vi "PH_IEEE1394Camera.get Cam Attribute.vi"(0 "IMAQ1394 Session In":T4, 1 "Cam Attribute Name":string, 2 "Attribute Information Array":T3(array[cluster]), 5 "Cam Error in":errorcluster) -> (14 "IMAQ1394 Session Out":T4, 15 "Attribute read?":bool, 16 "Cam Attribute Value":T1, 19 "Cam Error out":errorcluster)   [LabVIEW 2014, in "PH_IEEE1394Camera.lvlib"]
doc: "This VI gets a camera attribute."
uses:
  PH_IEEE1394Camera.lvlib
  <vilib>/userdefined/High Color/IMAQdx.ctl
  <vilib>/vision/driver/IMAQdx.llb/IMAQdx Attribute Type.ctl
  PH_IEEE1394Camera.Cam Attribute.ctl
  <resource>/objmgr/imaqdx.rc
  <vilib>/vision/driver/NI_Vision_Acquisition_Software.lvlib
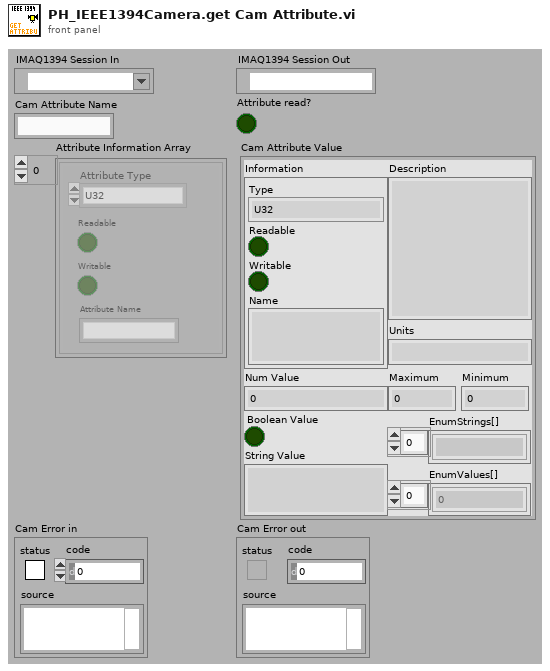
[diagram p1: front panel]
types:
  T1 = typedef "PH_IEEE1394Camera.lvlib/PH_IEEE1394Camera.Cam Attribute.ctl" = cluster{"Information":cluster{"Type":T2, "Readable":bool, "Writable":bool, "Name":string}, "Num Value":dbl, "String Value":string, "Maximum":dbl, "Minimum":dbl, "Units":string, "Description":string, "EnumStrings[]":string[], "EnumValues[]":u32[], "Boolean Value":bool}
  T2 = typedef "NI_Vision_Acquisition_Software.lvlib/IMAQdx Attribute Type.ctl" = enum32{"U32", "I64", "DBL", "String", "Enum", "Bool", "Command"}
  T3 = cluster{"Attribute Type":T2, "Readable":bool, "Writable":bool, "Attribute Name":string}[]
  T4 = typedef "IMAQdx.ctl" = refnum<k21>
  T5 = cluster{"Attribute Type":T2, "Readable":bool, "Writable":bool, "Attribute Name":string}
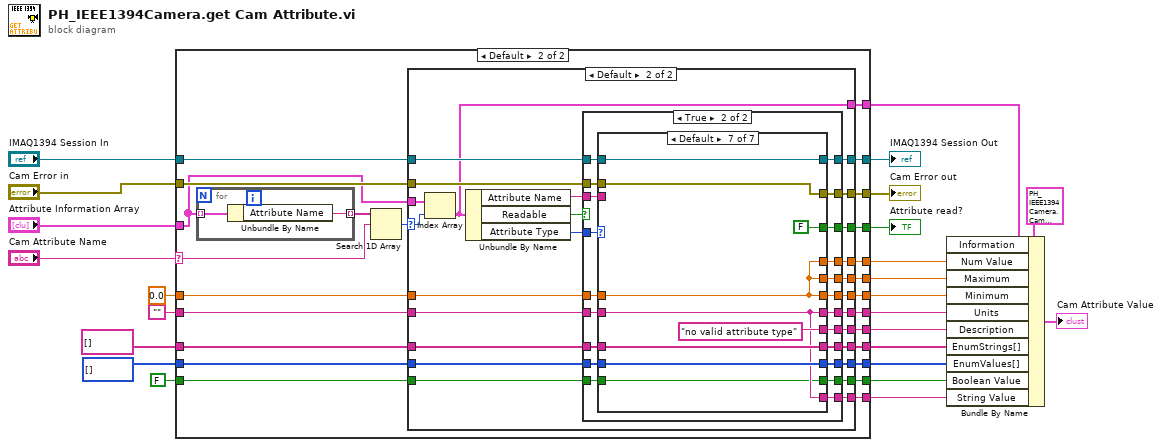
[diagram p0: block diagram]
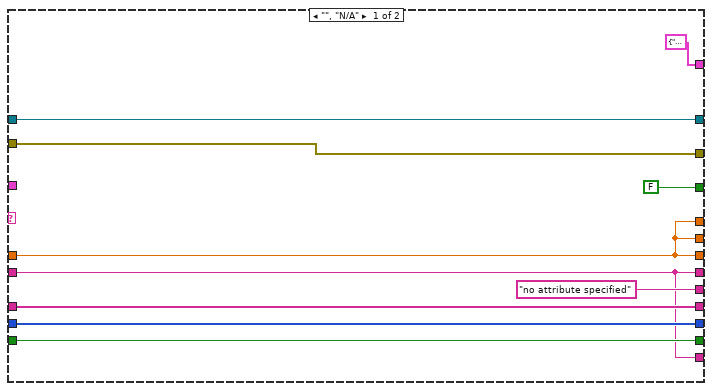
[diagram p2: hidden frame]
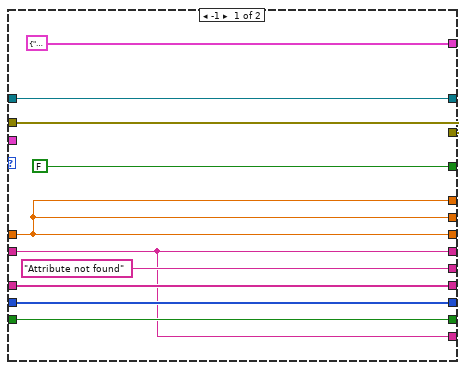
[diagram p3: hidden frame]
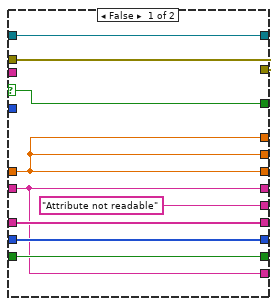
[diagram p4: hidden frame]
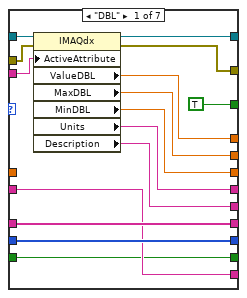
[diagram p5: hidden frame]
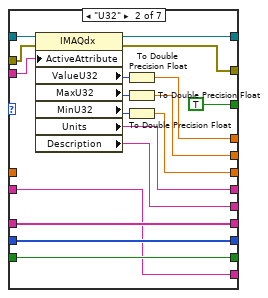
[diagram p6: hidden frame]
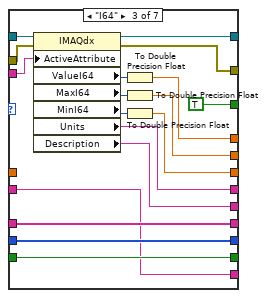
[diagram p7: hidden frame]
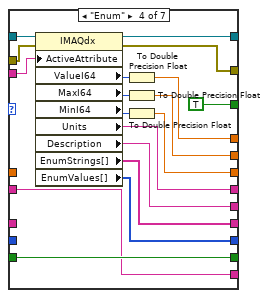
[diagram p8: hidden frame]
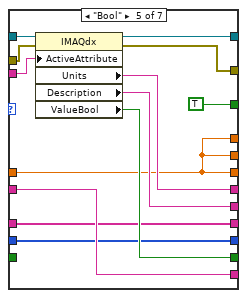
[diagram p9: hidden frame]
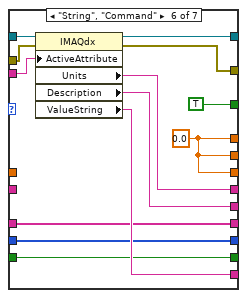
[diagram p10: hidden frame]
diagram:
  n1 = case shown="Default" "Cam Attribute Name" {
    selector: "Cam Attribute Name" -> [_ w54]
    tunnel: [w34 w58] -> w24
    tunnel: [w33 w57] -> w23
    tunnel: "Cam Error in" -> [w33 w56]
    tunnel: "IMAQ1394 Session In" -> [w34 w53]
    tunnel: [FALSE w55] -> w20
    tunnel: [w29 w52] -> w15
    tunnel: [w29 w51] -> w14
    tunnel: [w29 w50] -> w13
    tunnel: [w25 w49] -> w12
    tunnel: ["no attribute specified" w48] -> w11
    tunnel: [w28 w47] -> w10
    tunnel: [w27 w46] -> w9
    tunnel: [w26 w45] -> w8
    tunnel: [w25 w44] -> w7
    tunnel: "Attribute Information Array" -> [_ w43]
    tunnel: [T5 {"Attribute Type"=enum."U32", "Readable"=FALSE, "Writable"=FALSE, "Attribute Name"=""} ("Attribute Information") w40] -> w16
    tunnel: 0.0 ("ValueDBL") -> [w29 w39]
    tunnel: "" -> [w25 w38]
    tunnel: string[] [] ("EnumStrings[] 2") -> [w28 w37]
    tunnel: u32[] [] ("EnumValues[]") -> [w27 w36]
    tunnel: FALSE ("ValueBool") -> [w26 w35]
    frame "", "N/A" {
    }
    frame Default {
      n2 = for {
        tunnel: w43 -> [w229] mode=indexing
        tunnel: [w228] -> w42 mode=indexing
        n3 = Unbundle By Name(w229) -> ("Attribute Name"=w228:string)
      }
      n4 = Search 1D Array(1D array=w42, element=w54) -> (index of element=w41:i32)  [unwired: 1 in]
      n5 = case shown="Default" w41 {
        selector: w41 -> [_ w88]
        tunnel: [w67 w93] -> w58
        tunnel: w56 -> [w68 w92]
        tunnel: [w68 w91] -> w57
        tunnel: w53 -> [w67 w90]
        tunnel: w43 -> [_ w89]
        tunnel: [FALSE w85] -> w55
        tunnel: [w64 w83] -> w52
        tunnel: [w64 w82] -> w51
        tunnel: [w64 w81] -> w50
        tunnel: [w59 w80] -> w49
        tunnel: ["Attribute not found" w79] -> w48
        tunnel: [w62 w78] -> w47
        tunnel: [w61 w77] -> w46
        tunnel: [w60 w76] -> w45
        tunnel: [w59 w75] -> w44
        tunnel: [T5 {"Attribute Type"=enum."U32", "Readable"=FALSE, "Writable"=FALSE, "Attribute Name"=""} ("Attribute Information") w74] -> w40
        tunnel: w37 -> [w62 w73]
        tunnel: w36 -> [w61 w72]
        tunnel: w38 -> [w59 w71]
        tunnel: w39 -> [w64 w70]
        tunnel: w35 -> [w60 w69]
        frame -1 {
        }
        frame Default {
          n6 = Index Array(array=w89, index=w88) -> (element=w74:T5)
          n7 = Unbundle By Name(w74) -> ("Attribute Name"=w87:string, "Readable"=w86:bool, "Attribute Type"=w84:T2)
          n8 = case shown="True" w86 {
            selector: w86 -> [w100 _]
            tunnel: [w102 w123] -> w93
            tunnel: w92 -> [w101 w122]
            tunnel: [w101 w121] -> w91
            tunnel: w90 -> [w102 w120]
            tunnel: w87 -> [_ w119]
            tunnel: [w100 w118] -> w85
            tunnel: w84 -> [_ w113]
            tunnel: [w98 w117] -> w83
            tunnel: [w98 w116] -> w82
            tunnel: [w98 w115] -> w81
            tunnel: [w94 w114] -> w80
            tunnel: ["Attribute not readable" w112] -> w79
            tunnel: [w97 w111] -> w78
            tunnel: [w96 w110] -> w77
            tunnel: [w95 w109] -> w76
            tunnel: [w94 w108] -> w75
            tunnel: w70 -> [w98 w107]
            tunnel: w71 -> [w94 w106]
            tunnel: w72 -> [w96 w105]
            tunnel: w73 -> [w97 w104]
            tunnel: w69 -> [w95 w103]
            frame False {
            }
            frame True {
              n9 = case shown="Default" w113 {
                tunnel: [w138 w156 w174 w192 w205 w218 w226] -> w123
                tunnel: w122 -> [w134 w152 w170 w188 w201 w214 w225]
                tunnel: [w137 w155 w173 w191 w204 w217 w225] -> w121
                tunnel: w120 -> [w135 w153 w171 w189 w202 w215 w226]
                tunnel: w119 -> [w136 w154 w172 w190 w203 w216 _]
                tunnel: [TRUE TRUE TRUE TRUE TRUE TRUE FALSE] -> w118
                tunnel: [w130 w145 w163 w179 w193 w209 w223] -> w117
                tunnel: [w128 w144 w162 w178 w193 w209 w223] -> w116
                tunnel: [w129 w143 w161 w177 w193 w209 w223] -> w115
                tunnel: [w132 w150 w168 w186 w199 w212 w220] -> w114
                tunnel: [w131 w149 w167 w185 w198 w211 "no valid attribute type" ("Description")] -> w112
                tunnel: [w127 w142 w160 w181 w195 w208 w221] -> w111
                tunnel: [w126 w141 w159 w180 w194 w207 w222] -> w110
                tunnel: [w124 w140 w158 w176 w197 w206 w219] -> w109
                tunnel: [w125 w139 w157 w175 w196 w210 w220] -> w108
                tunnel: w107 -> [_ _ _ _ w193 _ w223]
                tunnel: w106 -> [w125 w139 w157 w175 w196 _ w220]
                tunnel: w105 -> [w126 w141 w159 _ w194 w207 w222]
                tunnel: w104 -> [w127 w142 w160 _ w195 w208 w221]
                tunnel: w103 -> [w124 w140 w158 w176 _ w206 w219]
                frame "DBL" {
                  n10 = property class="IMAQdx"(reference=w135, error in=w134, "ActiveAttribute"=w136) -> (reference out=w138:T4, error out=w137:errorcluster, "ValueDBL"=w130:dbl, "MaxDBL"=w128:dbl, "MinDBL"=w129:dbl, "Units"=w132:string, "Description"=w131:string)
                }
                frame "U32" {
                  n11 = property class="IMAQdx"(reference=w153, error in=w152, "ActiveAttribute"=w154) -> (reference out=w156:T4, error out=w155:errorcluster, "ValueU32"=w148:u32, "MaxU32"=w146:u32, "MinU32"=w147:u32, "Units"=w150:string, "Description"=w149:string)
                  n12 = To Double Precision Float(number=w148) -> (double precision float=w145:dbl)
                  n13 = To Double Precision Float(number=w146) -> (double precision float=w144:dbl)
                  n14 = To Double Precision Float(number=w147) -> (double precision float=w143:dbl)
                }
                frame "I64" {
                  n15 = property class="IMAQdx"(reference=w171, error in=w170, "ActiveAttribute"=w172) -> (reference out=w174:T4, error out=w173:errorcluster, "ValueI64"=w166:i64, "MaxI64"=w164:i64, "MinI64"=w165:i64, "Units"=w168:string, "Description"=w167:string)
                  n16 = To Double Precision Float(number=w166) -> (double precision float=w163:dbl)
                  n17 = To Double Precision Float(number=w164) -> (double precision float=w162:dbl)
                  n18 = To Double Precision Float(number=w165) -> (double precision float=w161:dbl)
                }
                frame "Enum" {
                  n19 = property class="IMAQdx"(reference=w189, error in=w188, "ActiveAttribute"=w190) -> (reference out=w192:T4, error out=w191:errorcluster, "ValueI64"=w184:i64, "MaxI64"=w182:i64, "MinI64"=w183:i64, "Units"=w186:string, "Description"=w185:string, "EnumStrings[]"=w181:string[], "EnumValues[]"=w180:u32[])
                  n20 = To Double Precision Float(number=w184) -> (double precision float=w179:dbl)
                  n21 = To Double Precision Float(number=w182) -> (double precision float=w178:dbl)
                  n22 = To Double Precision Float(number=w183) -> (double precision float=w177:dbl)
                }
                frame "Bool" {
                  n23 = property class="IMAQdx"(reference=w202, error in=w201, "ActiveAttribute"=w203) -> (reference out=w205:T4, error out=w204:errorcluster, "Units"=w199:string, "Description"=w198:string, "ValueBool"=w197:bool)
                }
                frame "String", "Command" {
                  w209 = 0.0 ("ValueDBL")
                  n24 = property class="IMAQdx"(reference=w215, error in=w214, "ActiveAttribute"=w216) -> (reference out=w218:T4, error out=w217:errorcluster, "Units"=w212:string, "Description"=w211:string, "ValueString"=w210:string)
                }
                frame Default {
                }
              }
            }
          }
        }
      }
    }
  }
  "Cam Error out" <- w23
  "Attribute read?" <- w20
  "IMAQ1394 Session Out" <- w24
  n25 = Bundle By Name(cluster=T1 {"Information"={"Type"=enum."U32", "Readable"=FALSE, "Writable"=FALSE, "Name"=""}, "Num Value"=0.0, "String Value"="", "Maximum"=0.0, "Minimum"=0.0, "Units"="", "Description"="", "EnumStrings[]"=[], "EnumValues[]"=[], "Boolean Value"=FALSE} ("Attribute"), "Information"=w16, "Num Value"=w15, "Maximum"=w14, "Minimum"=w13, "Units"=w12, "Description"=w11, "EnumStrings[]"=w10, "EnumValues[]"=w9, "Boolean Value"=w8, "String Value"=w7) -> (→"Cam Attribute Value":T1)
